vi "Main.vi"() -> ()   [LabVIEW 2017]
uses:
  controls_main.ctl
  EventQueueCluster.ctl
  EventMessage.ctl
  GUIQueueCluster.ctl
  GUIMessage.ctl
  MeasureQueue.ctl
  MeasureMessage.ctl
  HardwareQueueCluster.ctl
  hardwareMessage.ctl
  SaveQueueCluster.ctl
  SaveMessage.ctl
panel:
  in  "Save Data":bool
  in  "Clean error":bool
  in  "Error description":string
  in  "Phys.channel 3":dbl=2.0
  in  "Phys.channel 2":dbl=1.0
  in  "Phys.channel 1":dbl
  in  "Arduino VISA resource name":refnum<visa-resource-name>
  in  "stop":bool
  in  "Ch3On":bool
  in  "Ch2On":bool
  in  "Ch1On":bool
  in  "R 3, kOhm":dbl=98.0
  in  "R 2, kOhm":dbl=98.0
  in  "R 1, kOhm":dbl=98.0
  out "Channel 3":dbl(slide) scale=0.0..150.0
  out "Channel 2":dbl(slide) scale=0.0..150.0
  out "Channel 1":dbl(slide) scale=0.0..150.0
  # "THERMISTORS TEMPERATURE"
  # "Channel 1"
  # "Channel 2"
  # "Channel 3"
  # "C"
  # "C"
  # "C"
  # "Excitonics lab. 2019. Michael Shustov"
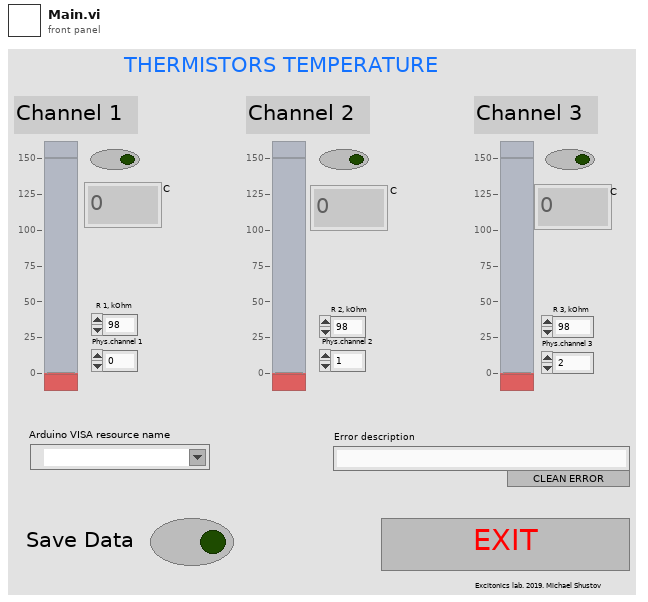
[diagram p1: front panel]
types:
  T1 = typedef "controls_main.ctl" = cluster{"stop":refnum<vi>, "Ch3On":refnum<vi>, "Ch2On":refnum<vi>, "Ch1On":refnum<vi>, "VISA resource name":refnum<vi>, "Phys.channel 3":refnum<vi>, "Phys.channel 2":refnum<vi>, "Phys.channel 1":refnum<vi>, "R 3, kOhm":refnum<vi>, "R 2, kOhm":refnum<vi>, "R 1, kOhm":refnum<vi>, "Channel 3":refnum<vi>, "Channel 2":refnum<vi>, "Channel 1":refnum<vi>, "Clean error":refnum<vi>, "Error description":refnum<vi>, "Path to save":refnum<vi>, "Save Data":refnum<vi>}
  T2 = typedef "QueueCluster.ctl" = cluster{"EventQueue":refnum<queue>, "MeasureQueue":refnum<queue>, "HardwareQueue":refnum<queue>, "GUIQueue":refnum<queue>, "SaveQueue":refnum<queue>}
  T3 = typedef "EventQueueCluster.ctl" = cluster{"EventsMessage":T4, "NumericValue":dbl, "String":string}
  T4 = typedef "EventMessage.ctl" = enum16{"Error", "Init", "Listen", "Halt"}
  T5 = typedef "GUIMessage.ctl" = enum16{"StopSave", "Channel1Value", "Channel2Value", "Channel3Value", "ErrorSource", "CleanError", "StartChannel1", "StartChannel2", "StartChannel3", "StopChannel1", "StopChannel2", "StopChannel3", "Halt"}
  T6 = typedef "GUIQueueCluster.ctl" = cluster{"GUIMessage":T5, "NumericValue":dbl, "String":string}
  T7 = typedef "MeasureQueue.ctl" = cluster{"NumericValue":dbl, "String":string, "MeasureMessage":T8}
  T8 = typedef "MeasureMessage.ctl" = enum16{"Init", "Measure", "Error", "Halt", "StartChannel", "StopChannel"}
  T9 = typedef "hardwareMessage.ctl" = enum16{"Init", "MeasureChannel", "CloseDevice", "Error", "Halt", "SetPhysChannel1", "SetPhysChannel2", "SetPhysChannel3"}
  T10 = typedef "HardwareQueueCluster.ctl" = cluster{"HardwareMessage":T9, "NumericValue":dbl, "String":string}
  T11 = typedef "SaveQueueCluster.ctl" = cluster{"Save message":T12, "NumericValue":dbl, "String":string}
  T12 = typedef "SaveMessage.ctl" = enum16{"StartSaving", "StopSaving", "Ch1Value", "Ch2Value", "Ch3Value", "Error", "WriteFile", "Halt"}
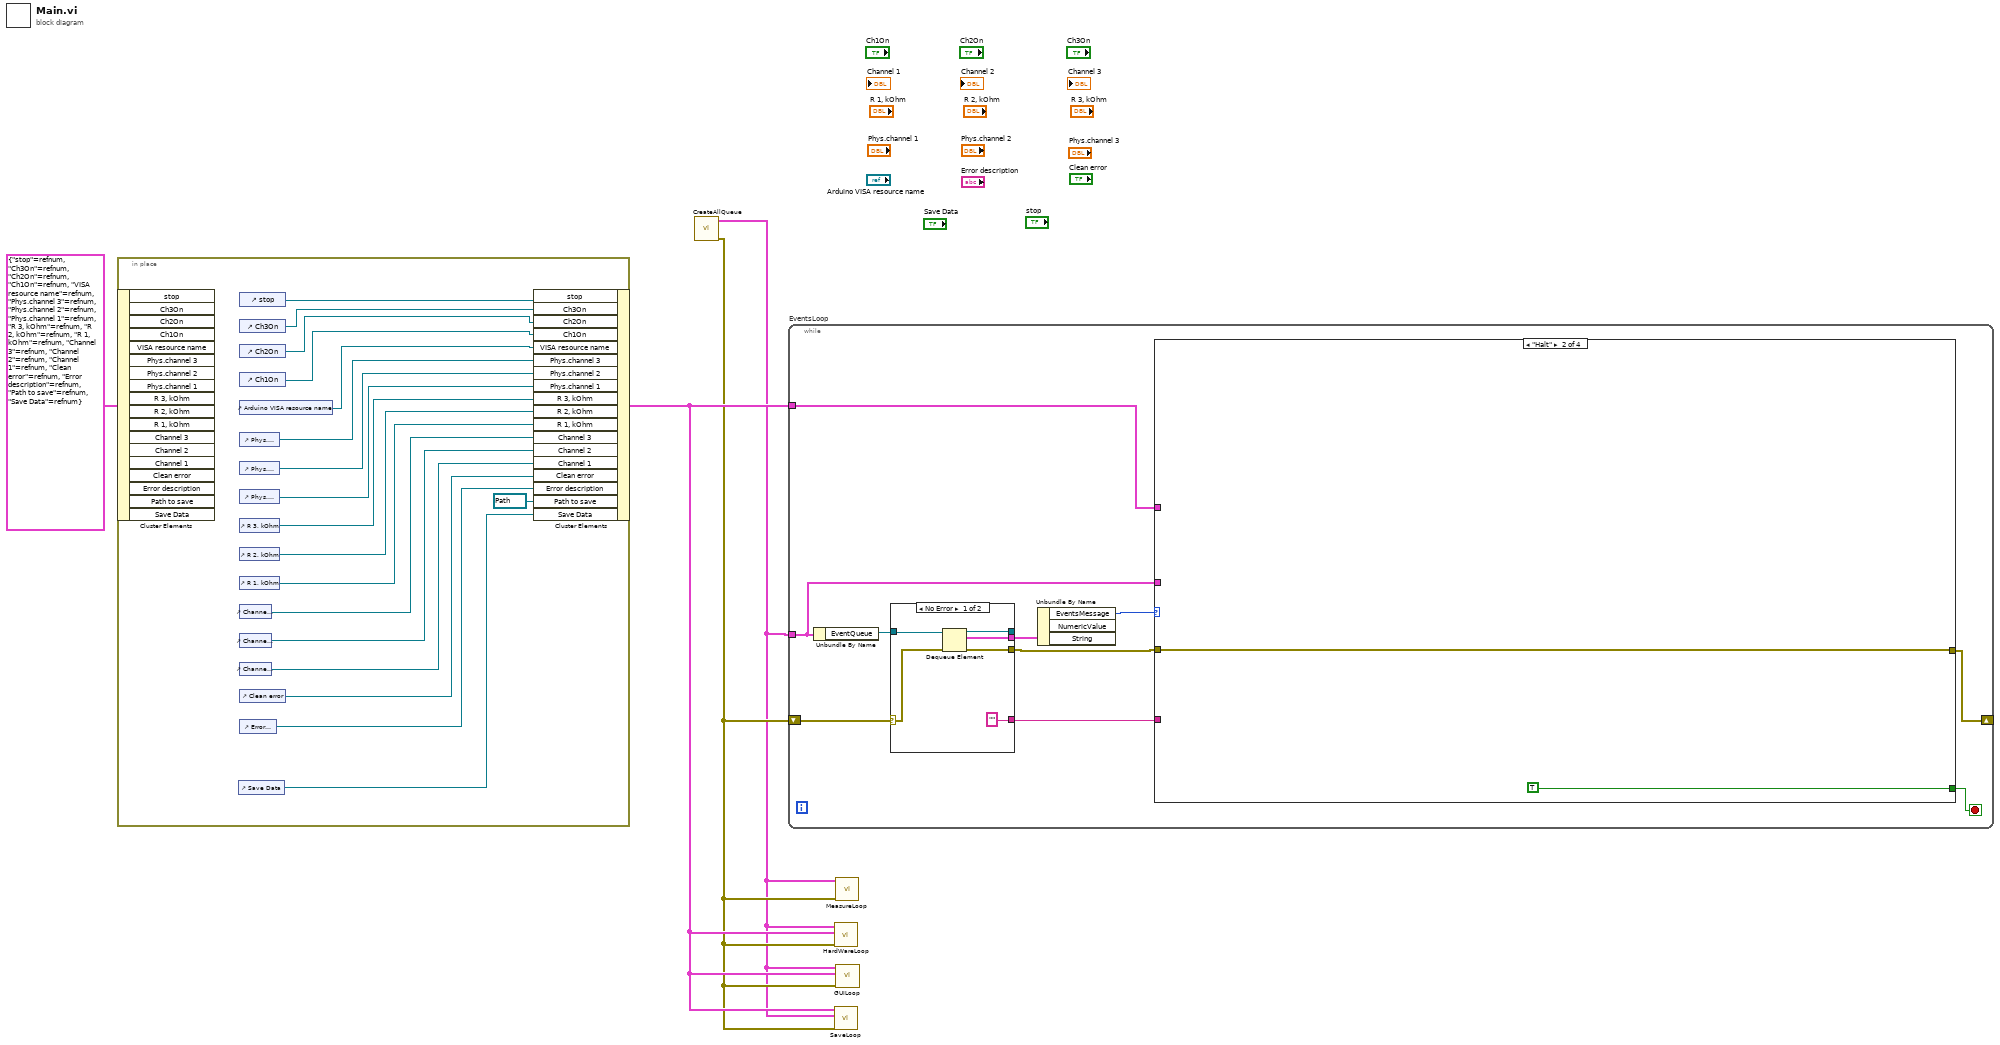
[diagram p0: block diagram]
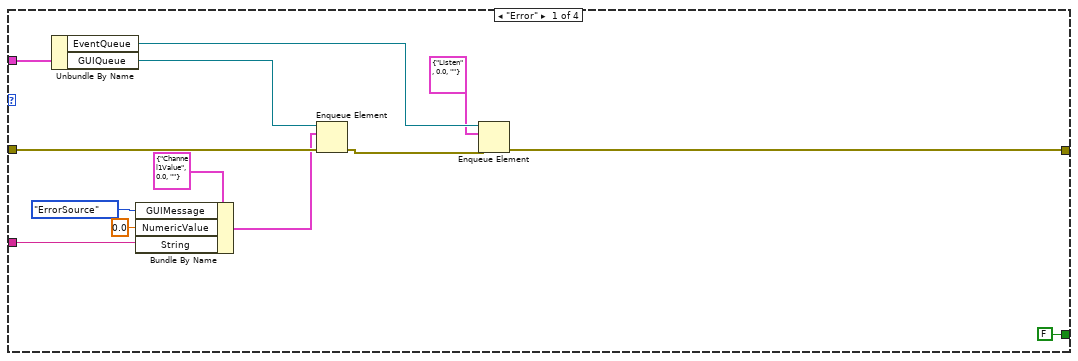
[diagram p2: hidden frame]
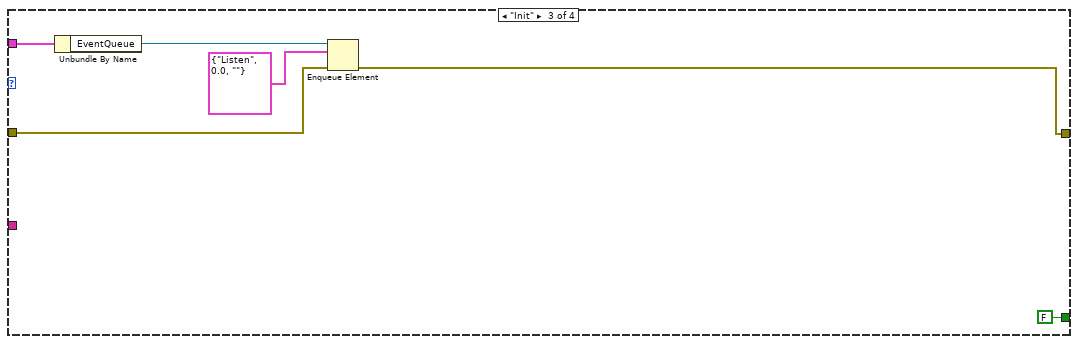
[diagram p3: hidden frame]
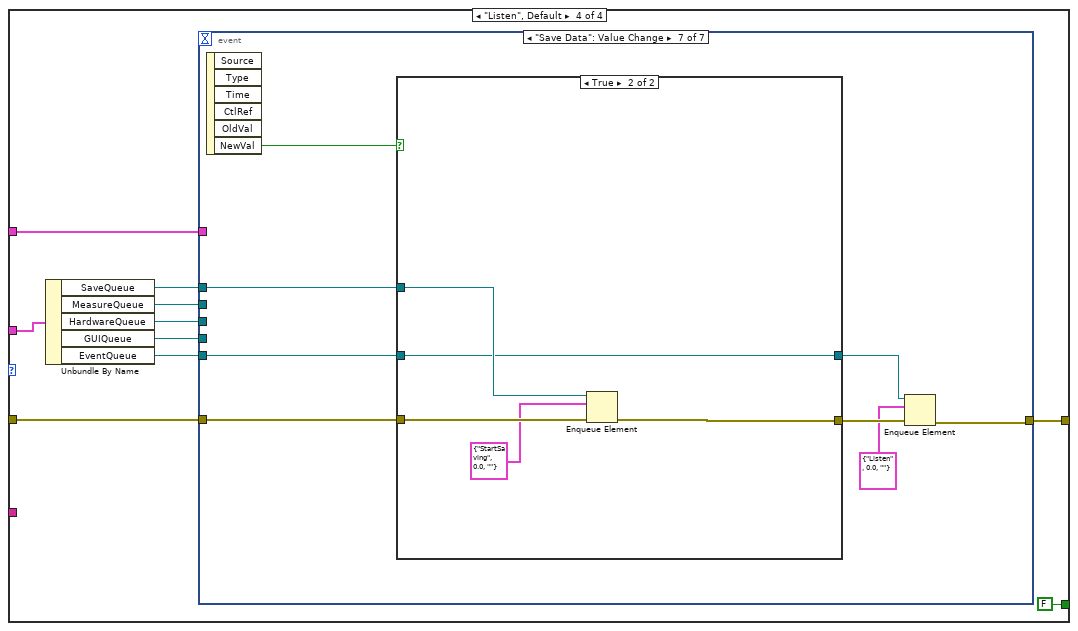
[diagram p4: hidden frame]
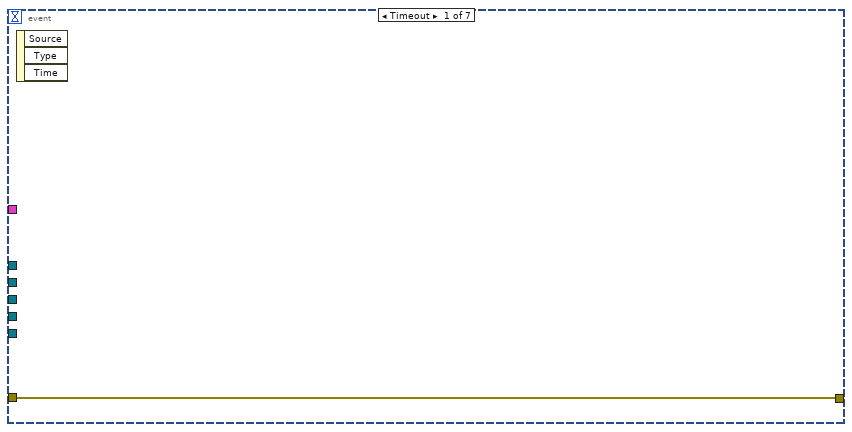
[diagram p5: hidden frame]
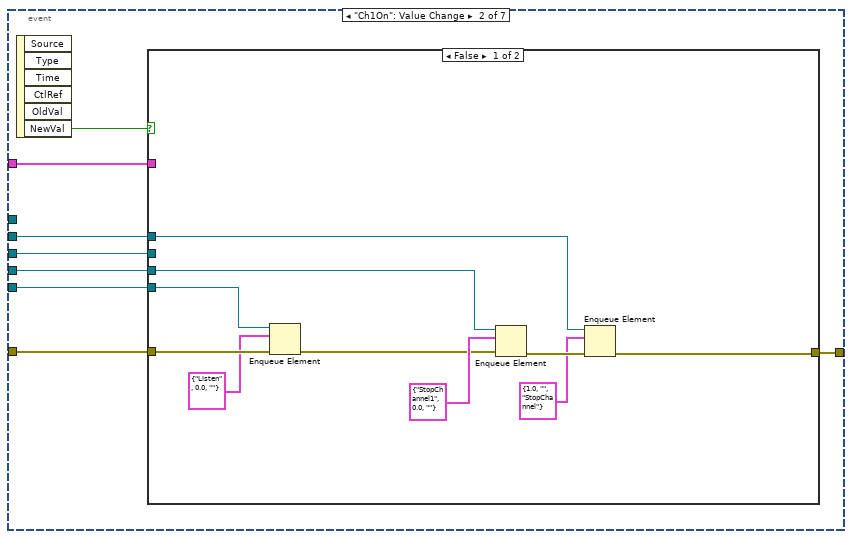
[diagram p6: hidden frame]
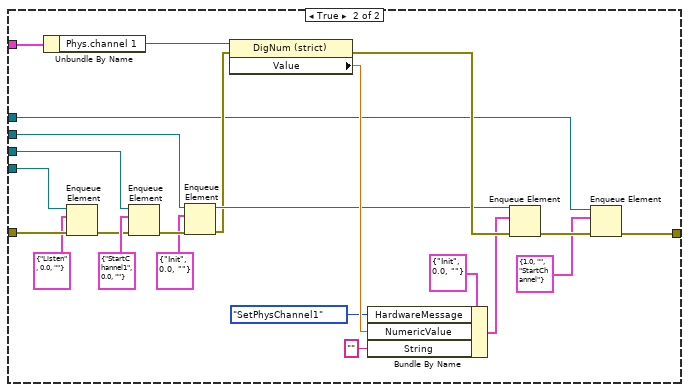
[diagram p7: hidden frame]
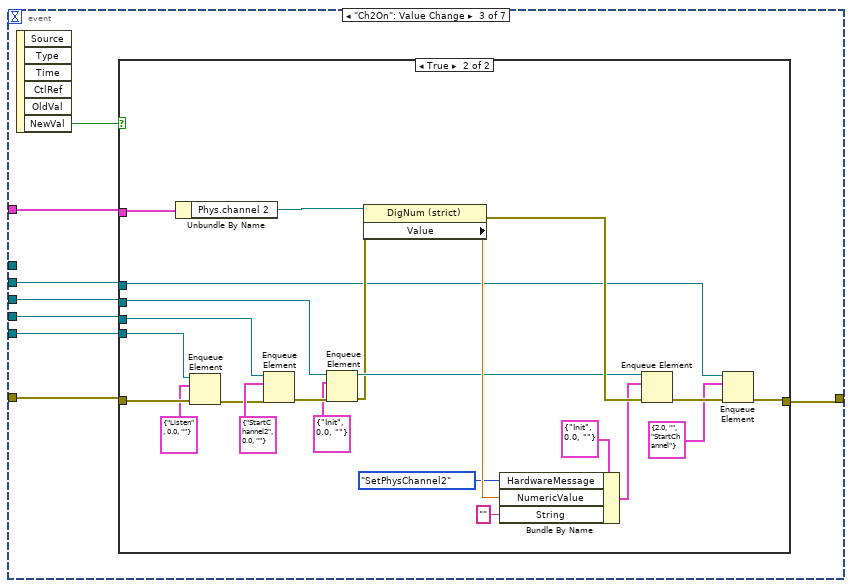
[diagram p8: hidden frame]
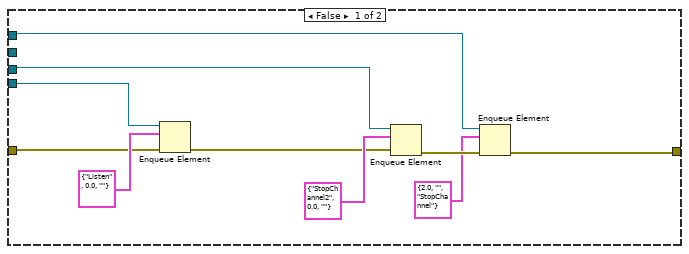
[diagram p9: hidden frame]
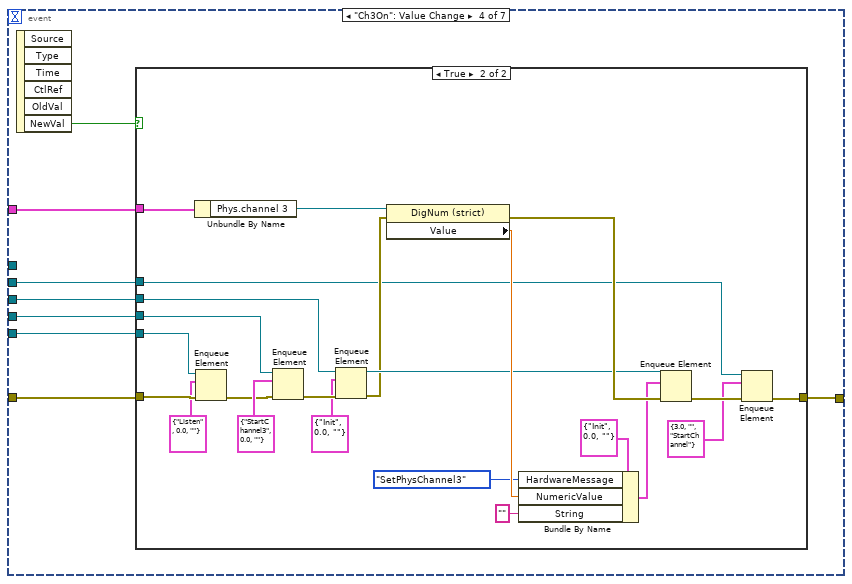
[diagram p10: hidden frame]
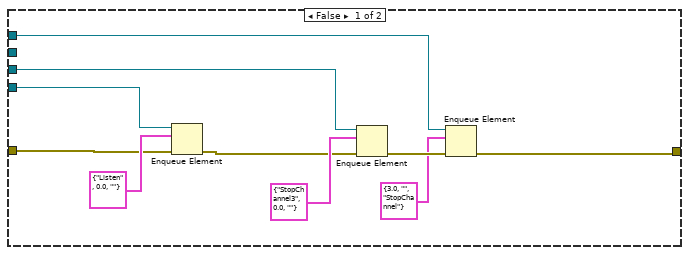
[diagram p11: hidden frame]
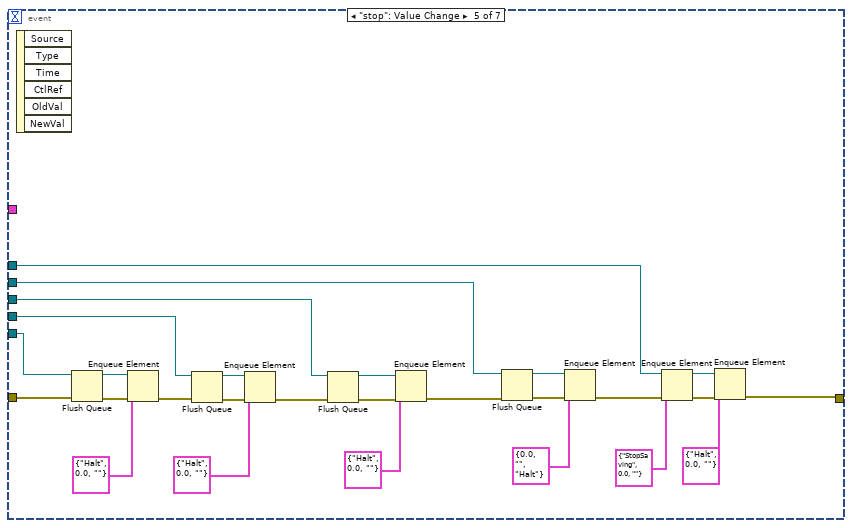
[diagram p12: hidden frame]
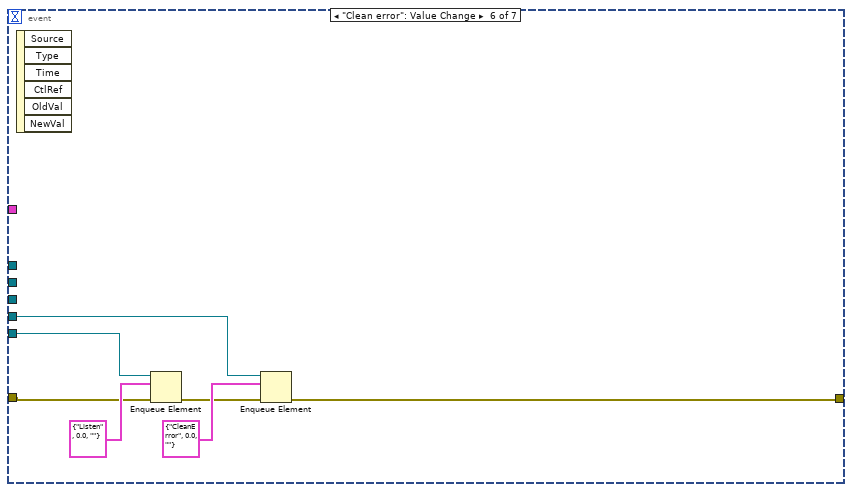
[diagram p13: hidden frame]
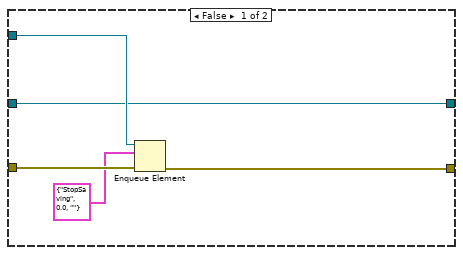
[diagram p14: hidden frame]
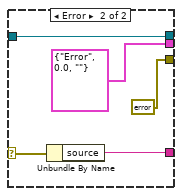
[diagram p15: hidden frame]
diagram:
  n1 = in-place {
    n2 = in-place-cluster #1(T1 {"stop"=refnum, "Ch3On"=refnum, "Ch2On"=refnum, "Ch1On"=refnum, "VISA resource name"=refnum, "Phys.channel 3"=refnum, "Phys.channel 2"=refnum, "Phys.channel 1"=refnum, "R 3, kOhm"=refnum, "R 2, kOhm"=refnum, "R 1, kOhm"=refnum, "Channel 3"=refnum, "Channel 2"=refnum, "Channel 1"=refnum, "Clean error"=refnum, "Error description"=refnum, "Path to save"=refnum, "Save Data"=refnum} ("ctrls")) -> ()  [unwired: 18 out]
    n3 = control-ref of="Save Data"() -> (w6:refnum<vi>)
    n4 = control-ref of="stop"() -> (w22:refnum<vi>)
    n5 = control-ref of="Ch3On"() -> (w21:refnum<vi>)
    n6 = control-ref of="Ch2On"() -> (w20:refnum<vi>)
    n7 = control-ref of="Ch1On"() -> (w19:refnum<vi>)
    n8 = control-ref of="Arduino VISA resource name"() -> (w18:refnum<vi>)
    n9 = control-ref of="Phys.channel 3"() -> (w17:refnum<vi>)
    n10 = control-ref of="Phys.channel 2"() -> (w16:refnum<vi>)
    n11 = control-ref of="Phys.channel 1"() -> (w15:refnum<vi>)
    n12 = control-ref of="R 3, kOhm"() -> (w14:refnum<vi>)
    n13 = control-ref of="R 2, kOhm"() -> (w13:refnum<vi>)
    n14 = control-ref of="R 1, kOhm"() -> (w12:refnum<vi>)
    n15 = control-ref of="Channel 3"() -> (w11:refnum<vi>)
    n16 = control-ref of="Channel 2"() -> (w10:refnum<vi>)
    n17 = control-ref of="Channel 1"() -> (w9:refnum<vi>)
    n18 = control-ref of="Clean error"() -> (w8:refnum<vi>)
    n19 = control-ref of="Error description"() -> (w7:refnum<vi>)
    n20 = in-place-cluster #1("stop"=w22, "Ch3On"=w21, "Ch2On"=w20, "Ch1On"=w19, "VISA resource name"=w18, "Phys.channel 3"=w17, "Phys.channel 2"=w16, "Phys.channel 1"=w15, "R 3, kOhm"=w14, "R 2, kOhm"=w13, "R 1, kOhm"=w12, "Channel 3"=w11, "Channel 2"=w10, "Channel 1"=w9, "Clean error"=w8, "Error description"=w7, "Path to save"=refnum<vi> refnum, "Save Data"=w6) -> (w3:T1)
  }
  n21 = call "CreateAllQueue.vi"() -> ("error out"=w2:errorcluster, "Queue cluster"=w1:T2)  [unwired: 10 in]
  n22 = while "EventsLoop" {
    tunnel: w3 -> [w25]
    shift-right: [w24] -> _
    shift-left: w2 -> [w29]
    tunnel: w1 -> [w23]
    stop <- w28 stop-if-true
    n23 = Unbundle By Name(w23) -> ("EventQueue"=w32:refnum<queue>)
    n24 = case shown="No Error" w29 {
      selector: w29 -> [w240 w248]
      tunnel: w32 -> [w245 w250]
      tunnel: [w244 w250] -> _
      tunnel: [w243 T3 {"EventsMessage"=enum."Error", "NumericValue"=0.0, "String"=""} ("EventQueueCluster")] -> w31
      tunnel: [w242 errorcluster {"status"=FALSE, "code"=0, "source"=""} ("error out")] -> w26
      tunnel: ["" ("source") w247] -> w27
      frame No Error {
        n25 = Dequeue Element(queue=w245, error in (no error)=w240) -> (queue out=w244:refnum<queue>, element=w243:T3, error out=w242:errorcluster)  [unwired: 1 in, 1 out]
      }
      frame Error {
        n26 = Unbundle By Name(w248) -> ("source"=w247:string)
      }
    }
    n27 = Unbundle By Name(w31) -> ("EventsMessage"=w30:T4)  [unwired: 2 out]
    n28 = case shown="\"Halt\"" w30 {
      tunnel: w27 -> [w42 _ _ _]
      tunnel: [FALSE TRUE FALSE FALSE] -> w28
      tunnel: w26 -> [w44 w46 w51 w59]
      tunnel: w25 -> [_ _ _ w58]
      tunnel: [w33 w46 w50 w57] -> w24
      tunnel: w23 -> [w37 _ w48 w55]
      frame "Error" {
        n29 = Unbundle By Name(w37) -> ("EventQueue"=w36:refnum<queue>, "GUIQueue"=w45:refnum<queue>)
        n30 = Bundle By Name(cluster=T6 {"GUIMessage"=enum."Channel1Value", "NumericValue"=0.0, "String"=""} ("element"), "GUIMessage"=GUIMessage."ErrorSource", "NumericValue"=0.0, "String"=w42) -> (w41:T6)
        n31 = Enqueue Element(queue=w45, element=w41, error in (no error)=w44) -> (error out=w35:errorcluster)  [unwired: 1 in, 2 out]
        n32 = Enqueue Element(queue=w36, element=T3 {"EventsMessage"=enum."Listen", "NumericValue"=0.0, "String"=""}, error in (no error)=w35) -> (error out=w33:errorcluster)  [unwired: 1 in, 2 out]
      }
      frame "Halt" {
      }
      frame "Init" {
        n33 = Unbundle By Name(w48) -> ("EventQueue"=w52:refnum<queue>)
        n34 = Enqueue Element(queue=w52, element=T3 {"EventsMessage"=enum."Listen", "NumericValue"=0.0, "String"=""}, error in (no error)=w51) -> (error out=w50:errorcluster)  [unwired: 1 in, 2 out]
      }
      frame "Listen", Default {
        n35 = Unbundle By Name(w55) -> ("SaveQueue"=w54:refnum<queue>, "MeasureQueue"=w63:refnum<queue>, "HardwareQueue"=w62:refnum<queue>, "GUIQueue"=w61:refnum<queue>, "EventQueue"=w60:refnum<queue>)
        n36 = event shown="[6] \"Save Data\": Value Change" {
          selector: _ -> [_ _ _ _ _ _ _]
          dyn-events: _ -> [_ _ _ _ _ _ _]
          timeout: _ -> [_ _ _ _ _ _ _]
          tunnel: w63 -> [_ w67 w111 w152 w202 _ _]
          tunnel: w62 -> [_ w69 w110 w151 w206 _ _]
          tunnel: w61 -> [_ w70 w109 w150 w210 w221 _]
          tunnel: w60 -> [_ w65 w106 w147 w213 w216 w223]
          tunnel: w59 -> [w64 w71 w108 w149 w214 w217 w227]
          tunnel: w58 -> [_ w68 w112 w154 _ _ _]
          tunnel: [w64 w66 w107 w148 w188 w220 w225] -> w57
          tunnel: w54 -> [_ _ _ _ w192 _ w228]
          event Timeout {
            n37 = event-data() -> ()  [unwired: 1 in, 3 out]
          }
          event "Ch1On": Value Change {
            n38 = event-data() -> ("NewVal"=w72:bool)  [unwired: 1 in, 5 out]
            n39 = case shown="False" w72 {
              tunnel: w71 -> [w76 w85]
              tunnel: w70 -> [w78 w105]
              tunnel: w69 -> [_ w103]
              tunnel: w68 -> [_ w102]
              tunnel: w67 -> [w79 w93]
              tunnel: [w77 w92] -> w66
              tunnel: w65 -> [w74 w86]
              frame False {
                n40 = Enqueue Element(queue=w74, element=T3 {"EventsMessage"=enum."Listen", "NumericValue"=0.0, "String"=""}, error in (no error)=w76) -> (error out=w75:errorcluster)  [unwired: 1 in, 2 out]
                n41 = Enqueue Element(queue=w78, element=T6 {"GUIMessage"=enum."StopChannel1", "NumericValue"=0.0, "String"=""}, error in (no error)=w75) -> (error out=w82:errorcluster)  [unwired: 1 in, 2 out]
                n42 = Enqueue Element(queue=w79, element=T7 {"NumericValue"=1.0, "String"="", "MeasureMessage"=enum."StopChannel"}, error in (no error)=w82) -> (error out=w77:errorcluster)  [unwired: 1 in, 2 out]
              }
              frame True {
                n43 = Unbundle By Name(w102) -> ("Phys.channel 1"=w101:refnum<vi>)
                n44 = Enqueue Element(queue=w86, element=T3 {"EventsMessage"=enum."Listen", "NumericValue"=0.0, "String"=""}, error in (no error)=w85) -> (error out=w84:errorcluster)  [unwired: 1 in, 2 out]
                n45 = Enqueue Element(queue=w105, element=T6 {"GUIMessage"=enum."StartChannel1", "NumericValue"=0.0, "String"=""}, error in (no error)=w84) -> (error out=w104:errorcluster)  [unwired: 1 in, 2 out]
                n46 = Enqueue Element(queue=w103, element=T10 {"HardwareMessage"=enum."Init", "NumericValue"=0.0, "String"=""}, error in (no error)=w104) -> (queue out=w96:refnum<queue>, error out=w95:errorcluster)  [unwired: 1 in, 1 out]
                n47 = property class="DigNum (strict)"(reference=w101, error in=w95) -> (error out=w100:errorcluster, "Value"=w98:dbl)  [unwired: 1 out]
                n48 = Bundle By Name(cluster=T10 {"HardwareMessage"=enum."Init", "NumericValue"=0.0, "String"=""} ("element"), "HardwareMessage"=hardwareMessage."SetPhysChannel1", "NumericValue"=w98, "String"="") -> (w97:T10)
                n49 = Enqueue Element(queue=w96, element=w97, error in (no error)=w100) -> (error out=w94:errorcluster)  [unwired: 1 in, 2 out]
                n50 = Enqueue Element(queue=w93, element=T7 {"NumericValue"=1.0, "String"="", "MeasureMessage"=enum."StartChannel"}, error in (no error)=w94) -> (error out=w92:errorcluster)  [unwired: 1 in, 2 out]
              }
            }
          }
          event "Ch2On": Value Change {
            n51 = event-data() -> ("NewVal"=w113:bool)  [unwired: 1 in, 5 out]
            n52 = case shown="True" w113 {
              tunnel: w108 -> [w116 w127]
              tunnel: w109 -> [w119 w132]
              tunnel: w110 -> [_ w131]
              tunnel: w112 -> [_ w129]
              tunnel: w111 -> [w120 w130]
              tunnel: [w118 w128] -> w107
              tunnel: w106 -> [w115 w125]
              frame False {
                n53 = Enqueue Element(queue=w115, element=T3 {"EventsMessage"=enum."Listen", "NumericValue"=0.0, "String"=""}, error in (no error)=w116) -> (error out=w114:errorcluster)  [unwired: 1 in, 2 out]
                n54 = Enqueue Element(queue=w119, element=T6 {"GUIMessage"=enum."StopChannel2", "NumericValue"=0.0, "String"=""}, error in (no error)=w114) -> (error out=w123:errorcluster)  [unwired: 1 in, 2 out]
                n55 = Enqueue Element(queue=w120, element=T7 {"NumericValue"=2.0, "String"="", "MeasureMessage"=enum."StopChannel"}, error in (no error)=w123) -> (error out=w118:errorcluster)  [unwired: 1 in, 2 out]
              }
              frame True {
                n56 = Unbundle By Name(w129) -> ("Phys.channel 2"=w145:refnum<vi>)
                n57 = Enqueue Element(queue=w125, element=T3 {"EventsMessage"=enum."Listen", "NumericValue"=0.0, "String"=""}, error in (no error)=w127) -> (error out=w126:errorcluster)  [unwired: 1 in, 2 out]
                n58 = Enqueue Element(queue=w132, element=T6 {"GUIMessage"=enum."StartChannel2", "NumericValue"=0.0, "String"=""}, error in (no error)=w126) -> (error out=w146:errorcluster)  [unwired: 1 in, 2 out]
                n59 = Enqueue Element(queue=w131, element=T10 {"HardwareMessage"=enum."Init", "NumericValue"=0.0, "String"=""}, error in (no error)=w146) -> (queue out=w140:refnum<queue>, error out=w139:errorcluster)  [unwired: 1 in, 1 out]
                n60 = property class="DigNum (strict)"(reference=w145, error in=w139) -> (error out=w144:errorcluster, "Value"=w142:dbl)  [unwired: 1 out]
                n61 = Bundle By Name(cluster=T10 {"HardwareMessage"=enum."Init", "NumericValue"=0.0, "String"=""} ("element"), "HardwareMessage"=hardwareMessage."SetPhysChannel2", "NumericValue"=w142, "String"="") -> (w141:T10)
                n62 = Enqueue Element(queue=w140, element=w141, error in (no error)=w144) -> (error out=w138:errorcluster)  [unwired: 1 in, 2 out]
                n63 = Enqueue Element(queue=w130, element=T7 {"NumericValue"=2.0, "String"="", "MeasureMessage"=enum."StartChannel"}, error in (no error)=w138) -> (error out=w128:errorcluster)  [unwired: 1 in, 2 out]
              }
            }
          }
          event "Ch3On": Value Change {
            n64 = event-data() -> ("NewVal"=w153:bool)  [unwired: 1 in, 5 out]
            n65 = case shown="True" w153 {
              tunnel: w149 -> [w157 w167]
              tunnel: w150 -> [w164 w170]
              tunnel: w151 -> [_ w171]
              tunnel: w154 -> [_ w173]
              tunnel: w152 -> [w162 w172]
              tunnel: [w161 w169] -> w148
              tunnel: w147 -> [w156 w166]
              frame False {
                n66 = Enqueue Element(queue=w156, element=T3 {"EventsMessage"=enum."Listen", "NumericValue"=0.0, "String"=""}, error in (no error)=w157) -> (error out=w155:errorcluster)  [unwired: 1 in, 2 out]
                n67 = Enqueue Element(queue=w164, element=T6 {"GUIMessage"=enum."StopChannel3", "NumericValue"=0.0, "String"=""}, error in (no error)=w155) -> (error out=w163:errorcluster)  [unwired: 1 in, 2 out]
                n68 = Enqueue Element(queue=w162, element=T7 {"NumericValue"=3.0, "String"="", "MeasureMessage"=enum."StopChannel"}, error in (no error)=w163) -> (error out=w161:errorcluster)  [unwired: 1 in, 2 out]
              }
              frame True {
                n69 = Unbundle By Name(w173) -> ("Phys.channel 3"=w186:refnum<vi>)
                n70 = Enqueue Element(queue=w166, element=T3 {"EventsMessage"=enum."Listen", "NumericValue"=0.0, "String"=""}, error in (no error)=w167) -> (error out=w168:errorcluster)  [unwired: 1 in, 2 out]
                n71 = Enqueue Element(queue=w170, element=T6 {"GUIMessage"=enum."StartChannel3", "NumericValue"=0.0, "String"=""}, error in (no error)=w168) -> (error out=w187:errorcluster)  [unwired: 1 in, 2 out]
                n72 = Enqueue Element(queue=w171, element=T10 {"HardwareMessage"=enum."Init", "NumericValue"=0.0, "String"=""}, error in (no error)=w187) -> (queue out=w181:refnum<queue>, error out=w180:errorcluster)  [unwired: 1 in, 1 out]
                n73 = property class="DigNum (strict)"(reference=w186, error in=w180) -> (error out=w185:errorcluster, "Value"=w183:dbl)  [unwired: 1 out]
                n74 = Bundle By Name(cluster=T10 {"HardwareMessage"=enum."Init", "NumericValue"=0.0, "String"=""} ("element"), "HardwareMessage"=hardwareMessage."SetPhysChannel3", "NumericValue"=w183, "String"="") -> (w182:T10)
                n75 = Enqueue Element(queue=w181, element=w182, error in (no error)=w185) -> (error out=w179:errorcluster)  [unwired: 1 in, 2 out]
                n76 = Enqueue Element(queue=w172, element=T7 {"NumericValue"=3.0, "String"="", "MeasureMessage"=enum."StartChannel"}, error in (no error)=w179) -> (error out=w169:errorcluster)  [unwired: 1 in, 2 out]
              }
            }
          }
          event "stop": Value Change {
            n77 = event-data() -> ()  [unwired: 1 in, 6 out]
            n78 = Flush Queue(queue=w213, error in (no error)=w214) -> (queue out=w211:refnum<queue>, error out=w212:errorcluster)  [unwired: 1 out]
            n79 = Enqueue Element(queue=w211, element=T3 {"EventsMessage"=enum."Halt", "NumericValue"=0.0, "String"=""}, error in (no error)=w212) -> (error out=w209:errorcluster)  [unwired: 1 in, 2 out]
            n80 = Flush Queue(queue=w210, error in (no error)=w209) -> (queue out=w208:refnum<queue>, error out=w207:errorcluster)  [unwired: 1 out]
            n81 = Enqueue Element(queue=w208, element=T6 {"GUIMessage"=enum."Halt", "NumericValue"=0.0, "String"=""}, error in (no error)=w207) -> (error out=w205:errorcluster)  [unwired: 1 in, 2 out]
            n82 = Flush Queue(queue=w206, error in (no error)=w205) -> (queue out=w204:refnum<queue>, error out=w203:errorcluster)  [unwired: 1 out]
            n83 = Enqueue Element(queue=w204, element=T10 {"HardwareMessage"=enum."Halt", "NumericValue"=0.0, "String"=""}, error in (no error)=w203) -> (error out=w201:errorcluster)  [unwired: 1 in, 2 out]
            n84 = Flush Queue(queue=w202, error in (no error)=w201) -> (queue out=w200:refnum<queue>, error out=w199:errorcluster)  [unwired: 1 out]
            n85 = Enqueue Element(queue=w200, element=T7 {"NumericValue"=0.0, "String"="", "MeasureMessage"=enum."Halt"}, error in (no error)=w199) -> (error out=w194:errorcluster)  [unwired: 1 in, 2 out]
            n86 = Enqueue Element(queue=w192, element=T11 {"Save message"=enum."StopSaving", "NumericValue"=0.0, "String"=""}, error in (no error)=w194) -> (queue out=w191:refnum<queue>, error out=w193:errorcluster)  [unwired: 1 in, 1 out]
            n87 = Enqueue Element(queue=w191, element=T11 {"Save message"=enum."Halt", "NumericValue"=0.0, "String"=""}, error in (no error)=w193) -> (error out=w188:errorcluster)  [unwired: 1 in, 2 out]
          }
          event "Clean error": Value Change {
            n88 = event-data() -> ()  [unwired: 1 in, 6 out]
            n89 = Enqueue Element(queue=w216, element=T3 {"EventsMessage"=enum."Listen", "NumericValue"=0.0, "String"=""}, error in (no error)=w217) -> (error out=w215:errorcluster)  [unwired: 1 in, 2 out]
            n90 = Enqueue Element(queue=w221, element=T6 {"GUIMessage"=enum."CleanError", "NumericValue"=0.0, "String"=""}, error in (no error)=w215) -> (error out=w220:errorcluster)  [unwired: 1 in, 2 out]
          }
          event "Save Data": Value Change {
            n91 = event-data() -> ("NewVal"=w229:bool)  [unwired: 1 in, 5 out]
            n92 = case shown="True" w229 {
              tunnel: w228 -> [w232 w239]
              tunnel: w227 -> [w234 w238]
              tunnel: [w233 w236] -> w226
              tunnel: [w230 w235] -> w224
              tunnel: w223 -> [w230 w235]
              frame False {
                n93 = Enqueue Element(queue=w232, element=T11 {"Save message"=enum."StopSaving", "NumericValue"=0.0, "String"=""}, error in (no error)=w234) -> (error out=w233:errorcluster)  [unwired: 1 in, 2 out]
              }
              frame True {
                n94 = Enqueue Element(queue=w239, element=T11 {"Save message"=enum."StartSaving", "NumericValue"=0.0, "String"=""}, error in (no error)=w238) -> (error out=w236:errorcluster)  [unwired: 1 in, 2 out]
              }
            }
            n95 = Enqueue Element(queue=w224, element=T3 {"EventsMessage"=enum."Listen", "NumericValue"=0.0, "String"=""}, error in (no error)=w226) -> (error out=w225:errorcluster)  [unwired: 1 in, 2 out]
          }
        }
      }
    }
  }
  n96 = call "HardWareLoop.vi"("error in (no error)"=w2, "ctrls"=w3, "Queue cluster"=w1) -> ()  [unwired: 9 in]
  n97 = call "SaveLoop.vi"("error in (no error)"=w2, "Queue cluster"=w1, "ctrls"=w3) -> ()  [unwired: 9 in]
  n98 = call "MeasureLoop.vi"("error in (no error)"=w2, "Queue cluster"=w1) -> ()  [unwired: 10 in]
  n99 = call "GUILoop.vi"("error in (no error)"=w2, "ctrls"=w3, "Queue cluster"=w1) -> ()  [unwired: 9 in]
